vi "GP307 Read.vi"(8 "error in":errorcluster, 11 "cRIO I/O Device":refnum<k21>="Mod7\\Port3") -> (0 "error out":errorcluster, 1 "Convectron 2":u8[](array[numeric]), 2 "Ion gauge 2":u8[](array[numeric]), 3 "Convectron 1":u8[](array[numeric]), 5 "Ion gauge 1":u8[](array[numeric]))   [LabVIEW 2016]
uses:
  <vilib>/rvi/eio/common/nirviEmuTemplateMethod_errors.vi
  <vilib>/eio/EIOMethodNode/EIOMethodNode.xnode
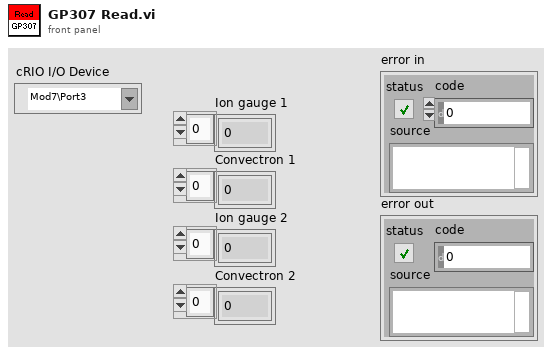
[diagram p1: front panel]
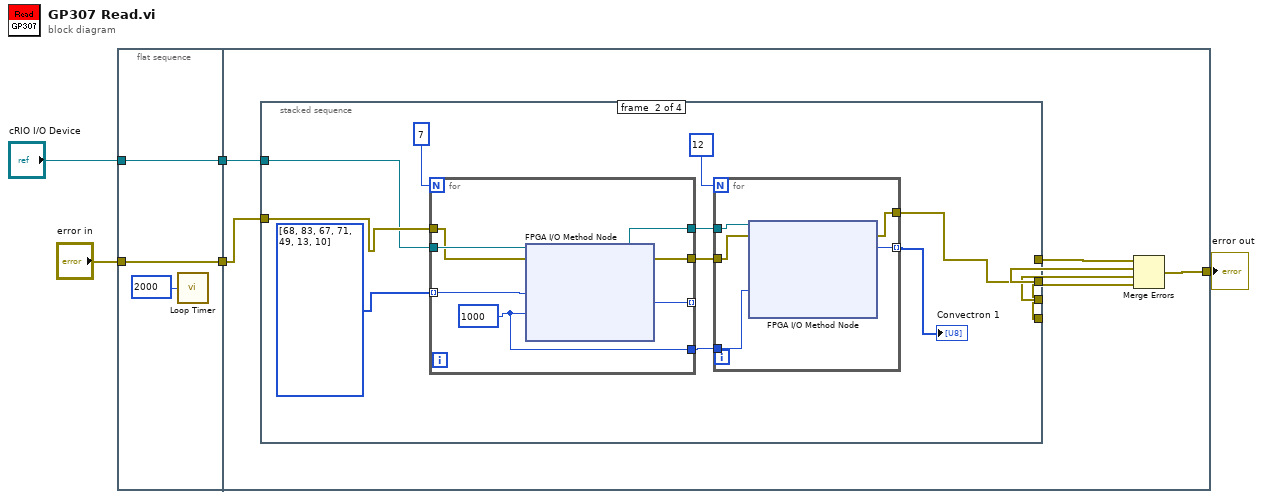
[diagram p0: block diagram]
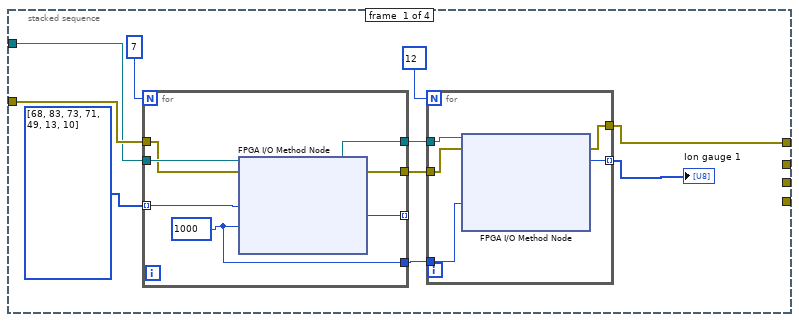
[diagram p2: hidden frame]
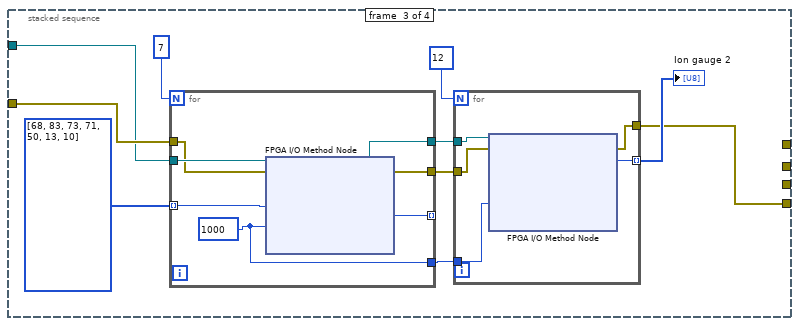
[diagram p3: hidden frame]
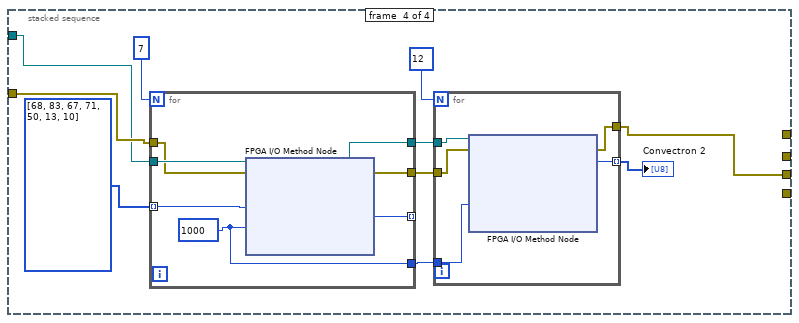
[diagram p4: hidden frame]
diagram:
  n1 = flat-sequence {
    tunnel: "error in" -> [w7]
    tunnel: [w7] -> w5
    tunnel: "cRIO I/O Device" -> [w6]
    tunnel: [w6] -> w1
    tunnel: w5 -> [w15]
    tunnel: [w13] -> w3
    tunnel: w1 -> [w9]
    frame #0 {
      n2 = call "Loop Timer"("Count(mSec)"=u32 2000 ("Count(Ticks)")) -> ()  [unwired: 1 out]
    }
    frame #1 {
      n3 = stacked-sequence {
        tunnel: w15 -> [w20 w40 w62 w81]
        tunnel: [w16 _ _ _] -> w14
        tunnel: [_ w37 _ _] -> w12
        tunnel: [_ _ _ w82] -> w11
        tunnel: [_ _ w60 _] -> w10
        tunnel: w9 -> [w18 w39 w59 w80]
        frame #0 {
          n4 = for {
            N: 7 -> [_]
            tunnel: [w34] -> w25
            tunnel: [w33] -> _ mode=indexing
            tunnel: u8[] [68, 83, 73, 71, 49, 13, 10] ("unsigned byte array") -> [w33] mode=indexing
            tunnel: w20 -> [w31]
            tunnel: [w36] -> w22
            tunnel: w18 -> [w35]
            tunnel: [w32] -> w21
            w34 = 1000 ("Timeout (ms)")
            n5 = xnode "FPGA I/O Method Node"("error in"=w31, "FPGA I/O In"=w35, "Data"=w33, "Timeout (ms)"=w34) -> ("error out"=w32:errorcluster, "FPGA I/O Out"=w36:refnum<k21>)  [unwired: 1 out]
          }
          n6 = for {
            N: 12 -> [_]
            tunnel: w25 -> [w27]
            tunnel: [w30] -> w17 mode=indexing
            tunnel: w22 -> [w29]
            tunnel: [w28] -> w16
            tunnel: w21 -> [w26]
            n7 = xnode "FPGA I/O Method Node"("error in"=w26, "FPGA I/O In"=w29, "Timeout (ms)"=w27) -> ("error out"=w28:errorcluster, "Data"=w30:u8)  [unwired: 2 out]
          }
          "Ion gauge 1" <- w17
        }
        frame #1 {
          n8 = for {
            N: 7 -> [_]
            tunnel: [w55] -> w46
            tunnel: [w54] -> _ mode=indexing
            tunnel: u8[] [68, 83, 67, 71, 49, 13, 10] ("unsigned byte array") -> [w54] mode=indexing
            tunnel: w40 -> [w52]
            tunnel: [w57] -> w43
            tunnel: w39 -> [w56]
            tunnel: [w53] -> w42
            w55 = 1000 ("Timeout (ms)")
            n9 = xnode "FPGA I/O Method Node"("error in"=w52, "FPGA I/O In"=w56, "Data"=w54, "Timeout (ms)"=w55) -> ("error out"=w53:errorcluster, "FPGA I/O Out"=w57:refnum<k21>)  [unwired: 1 out]
          }
          n10 = for {
            N: 12 -> [_]
            tunnel: w46 -> [w48]
            tunnel: [w51] -> w38 mode=indexing
            tunnel: w43 -> [w50]
            tunnel: [w49] -> w37
            tunnel: w42 -> [w47]
            n11 = xnode "FPGA I/O Method Node"("error in"=w47, "FPGA I/O In"=w50, "Timeout (ms)"=w48) -> ("error out"=w49:errorcluster, "Data"=w51:u8)  [unwired: 2 out]
          }
          "Convectron 1" <- w38
        }
        frame #2 {
          n12 = for {
            N: 7 -> [_]
            tunnel: [w76] -> w67
            tunnel: [w75] -> _ mode=indexing
            tunnel: u8[] [68, 83, 73, 71, 50, 13, 10] ("unsigned byte array") -> [w75] mode=indexing
            tunnel: w62 -> [w73]
            tunnel: [w78] -> w61
            tunnel: w59 -> [w77]
            tunnel: [w74] -> w58
            w76 = 1000 ("Timeout (ms)")
            n13 = xnode "FPGA I/O Method Node"("error in"=w73, "FPGA I/O In"=w77, "Data"=w75, "Timeout (ms)"=w76) -> ("error out"=w74:errorcluster, "FPGA I/O Out"=w78:refnum<k21>)  [unwired: 1 out]
          }
          n14 = for {
            N: 12 -> [_]
            tunnel: w67 -> [w69]
            tunnel: [w72] -> w63 mode=indexing
            tunnel: w61 -> [w71]
            tunnel: [w70] -> w60
            tunnel: w58 -> [w68]
            n15 = xnode "FPGA I/O Method Node"("error in"=w68, "FPGA I/O In"=w71, "Timeout (ms)"=w69) -> ("error out"=w70:errorcluster, "Data"=w72:u8)  [unwired: 2 out]
          }
          "Ion gauge 2" <- w63
        }
        frame #3 {
          n16 = for {
            N: 7 -> [_]
            tunnel: [w97] -> w88
            tunnel: [w96] -> _ mode=indexing
            tunnel: u8[] [68, 83, 67, 71, 50, 13, 10] ("unsigned byte array") -> [w96] mode=indexing
            tunnel: w81 -> [w94]
            tunnel: [w99] -> w85
            tunnel: w80 -> [w98]
            tunnel: [w95] -> w84
            w97 = 1000 ("Timeout (ms)")
            n17 = xnode "FPGA I/O Method Node"("error in"=w94, "FPGA I/O In"=w98, "Data"=w96, "Timeout (ms)"=w97) -> ("error out"=w95:errorcluster, "FPGA I/O Out"=w99:refnum<k21>)  [unwired: 1 out]
          }
          n18 = for {
            N: 12 -> [_]
            tunnel: w88 -> [w90]
            tunnel: [w93] -> w83 mode=indexing
            tunnel: w85 -> [w92]
            tunnel: [w91] -> w82
            tunnel: w84 -> [w89]
            n19 = xnode "FPGA I/O Method Node"("error in"=w89, "FPGA I/O In"=w92, "Timeout (ms)"=w90) -> ("error out"=w91:errorcluster, "Data"=w93:u8)  [unwired: 2 out]
          }
          "Convectron 2" <- w83
        }
      }
      n20 = Merge Errors(w14, w12, w11, w10) -> (w13:errorcluster)
    }
  }
  "error out" <- w3
